vi "Test EXE.vi"() -> ()   [LabVIEW 2019]
panel:
  out "Version":string
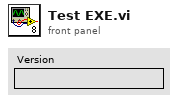
[diagram p1: front panel]
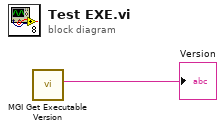
[diagram p0: block diagram]
diagram:
  n1 = call <userlib>:"MGI Get Executable Version.vi"() -> ("Version"=→"Version":string)  [unwired: 7 in]
